vi "GT Pvt Table Continuous.vi"(0 "cardNum":i16, 1 "tableId":i16, 2 "count":i32, 3 "pPos":dbl[](array[numeric]), 4 "pVel":dbl[](array[numeric]), 5 "pPercent":dbl[](array[numeric]), 6 "pVelMax":dbl[](array[numeric]), 7 "error in (no error)":errorcluster caption="错误输入（无错误）", 8 "pAcc":dbl[](array[numeric]), 9 "pDec":dbl[](array[numeric]), 10 "timeBegin":dbl) -> (18 "pAcc out":dbl[](array[numeric]), 19 "pDec out":dbl[](array[numeric]), 20 "function return":i16, 23 "pPos out":dbl[](array[numeric]), 24 "pVel out":dbl[](array[numeric]), 25 "pPercent out":dbl[](array[numeric]), 26 "pVelMax out":dbl[](array[numeric]), 27 "error out":errorcluster caption="错误输出")   [LabVIEW 2020, in "gts.lvlib"]
doc: "GT_API GT_PvtTableContinuous(short cardNum,short tableId,long count,double *pPos,double *pVel,double *pPercent,double *pVelMax,double *pAcc,double *pDec,double timeBegin);"
uses:
  gts.lvlib
  dll/32bit/multi_card/gts.dll
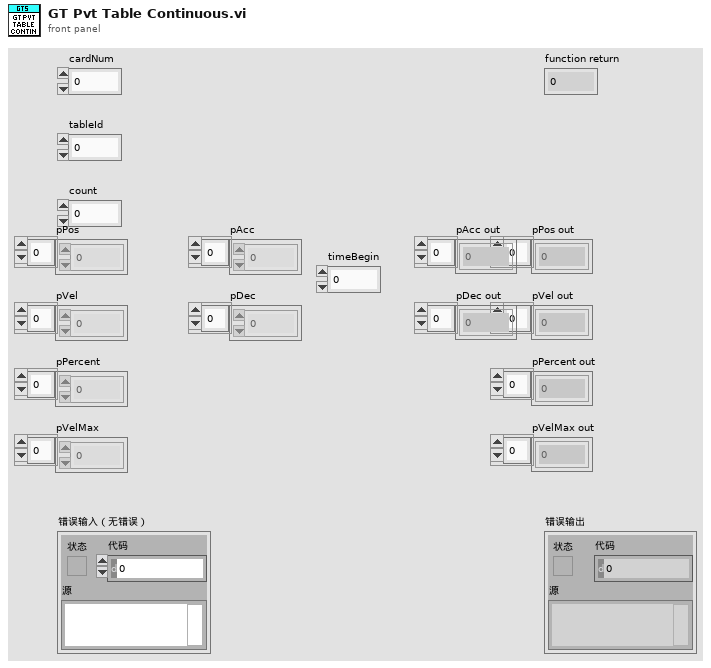
[diagram p1: front panel]
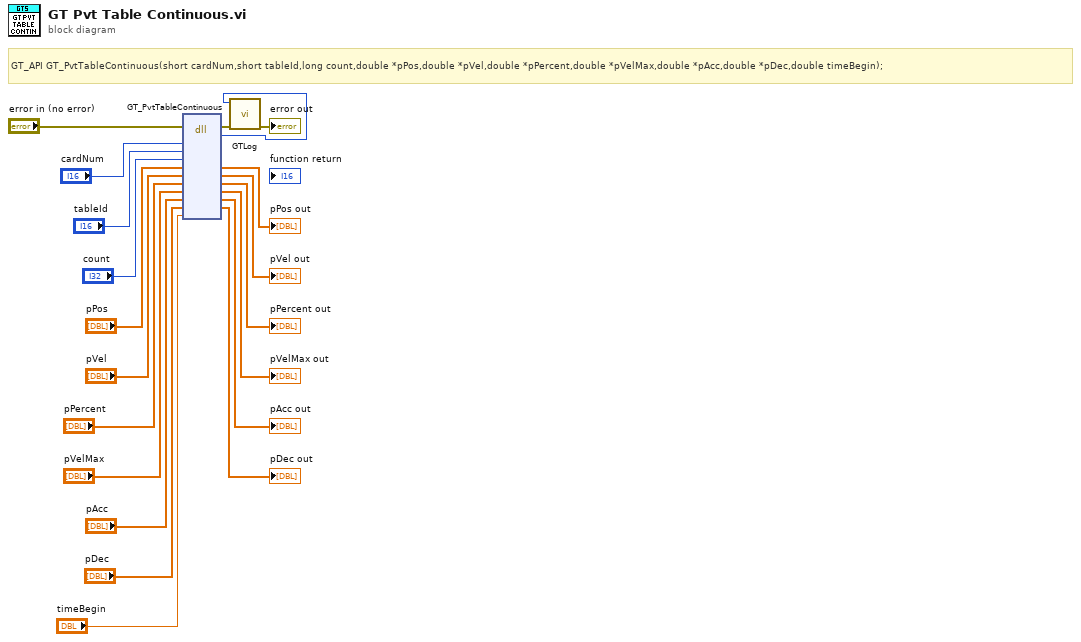
[diagram p0: block diagram]
diagram:
  # "GT_API GT_PvtTableContinuous(short cardNum,short tableId,long count,double *pPos,double *pVel,double *pPercent,double *pVelMax,double *pAcc,double *pDec,double timeBegin);"
  n1 = dll-call lib="C:/1228/dll/32bit/multi_card/gts.dll" fn="GT_PvtTableContinuous"(error in="error in (no error)", "cardNum"="cardNum", "tableId"="tableId", "count"="count", "pPos"="pPos", "pVel"="pVel", "pPercent"="pPercent", "pVelMax"="pVelMax", "pAcc"="pAcc", "pDec"="pDec", "timeBegin"="timeBegin") -> (error out=w3:errorcluster, "返回类型"=w1:i16, "pPos"=→"pPos out":dbl[], "pVel"=→"pVel out":dbl[], "pPercent"=→"pPercent out":dbl[], "pVelMax"=→"pVelMax out":dbl[], "pAcc"=→"pAcc out":dbl[], "pDec"=→"pDec out":dbl[])  [unwired: 6 in, 1 out]
  n2 = call "GTLog.vi"("error in (no error)"=w3, "Numeric"=w1) -> ("error out"=→"error out":errorcluster)  [unwired: 9 in]
